vi "Output_4ch_v00.vi"(8 "Outputs":T2, 11 "Safety First":T1) -> ()   [LabVIEW 2013]
doc: "Outputs the signals to FPGA output nodes, after a variable rate-limiter has been applied."
uses:
  Strict Type Defs/1SDI Output.ctl
  Strict Type Defs/Safety First.ctl
  <vilib>/rvi/eio/common/nirviEmuTemplateMethod_errors.vi
  <vilib>/rvi/Analysis/common/FxpNativeNode/niFpgaFxpNative.xnode
  <vilib>/eio/EIONode/EIONode.xnode
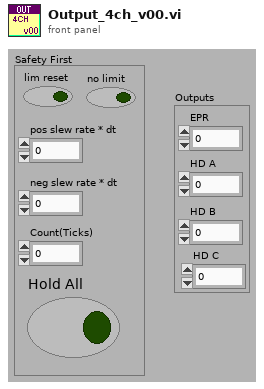
[diagram p1: front panel]
types:
  T1 = typedef "Safety First.ctl" = cluster{"lim reset":bool, "no limit":bool, "pos slew rate * dt":i16, "neg slew rate * dt":i16, "Hold All":bool, "Count(Ticks)":u32}
  T2 = typedef "1SDI Output.ctl" = cluster{"EPR":i16, "HD A":i16, "HD B":i16, "HD C":i16}
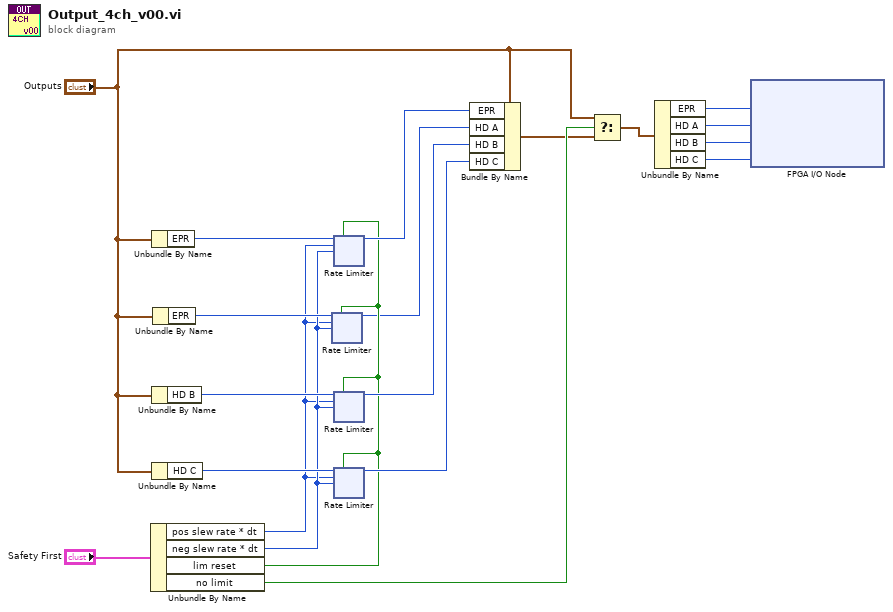
[diagram p0: block diagram]
diagram:
  n1 = Unbundle By Name("Safety First") -> ("pos slew rate * dt"=w3:i16, "neg slew rate * dt"=w4:i16, "lim reset"=w5:bool, "no limit"=w17:bool)
  n2 = Unbundle By Name("Outputs") -> ("EPR"=w19:i16)
  n3 = Unbundle By Name("Outputs") -> ("HD B"=w10:i16)
  n4 = Unbundle By Name("Outputs") -> ("HD C"=w11:i16)
  n5 = Unbundle By Name("Outputs") -> ("EPR"=w6:i16)
  n6 = xnode ("Rate Limiter")("pos slew rate * dt"=w3, "input"=w6, "neg slew rate * dt"=w4, "reset"=w5) -> ("output"=w2:i16)
  n7 = xnode ("Rate Limiter")("pos slew rate * dt"=w3, "input"=w19, "neg slew rate * dt"=w4, "reset"=w5) -> ("output"=w18:i16)
  n8 = xnode ("Rate Limiter")("pos slew rate * dt"=w3, "input"=w10, "neg slew rate * dt"=w4, "reset"=w5) -> ("output"=w8:i16)
  n9 = xnode ("Rate Limiter")("pos slew rate * dt"=w3, "input"=w11, "neg slew rate * dt"=w4, "reset"=w5) -> ("output"=w9:i16)
  n10 = Bundle By Name(cluster="Outputs", "EPR"=w18, "HD A"=w2, "HD B"=w8, "HD C"=w9) -> (w12:T2)
  n11 = Select(t="Outputs", s=w17, f=w12) -> (s? t:f=w16:T2)
  n12 = Unbundle By Name(w16) -> ("EPR"=w15:i16, "HD A"=w14:i16, "HD B"=w13:i16, "HD C"=w1:i16)
  n13 = xnode "FPGA I/O Node"("Connector0/AO0"=w15, "Connector0/AO1"=w14, "Connector0/AO2"=w13, "Connector0/AO3"=w1) -> ()  [unwired: 4 in, 4 out]
